vi "Call_signal_fromHW.vi"(5 "Plot window":string) -> (1 "Selected signals":string[](array[string]), 2 "Ready?":bool)   [LabVIEW 2022 SP3]
doc: "Through this function you can select the stored signals from the Main_menu."
panel:
  in  "Working Path":path
  in  "Load Signals profile":bool
  in  "Save Signals profile":bool
  in  "Select signals":i32[](listbox)
  out "Clone Name":string
  in  "Add to graph":bool
  # "First Save Signals before\nto load Signals"
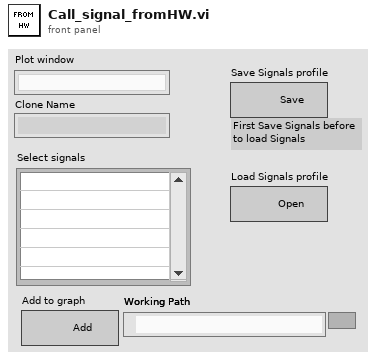
[diagram p1: front panel]
types:
  T1 = enum32{"Invalid", "Standard", "Closed", "Hidden", "Minimized", "Maximized"}
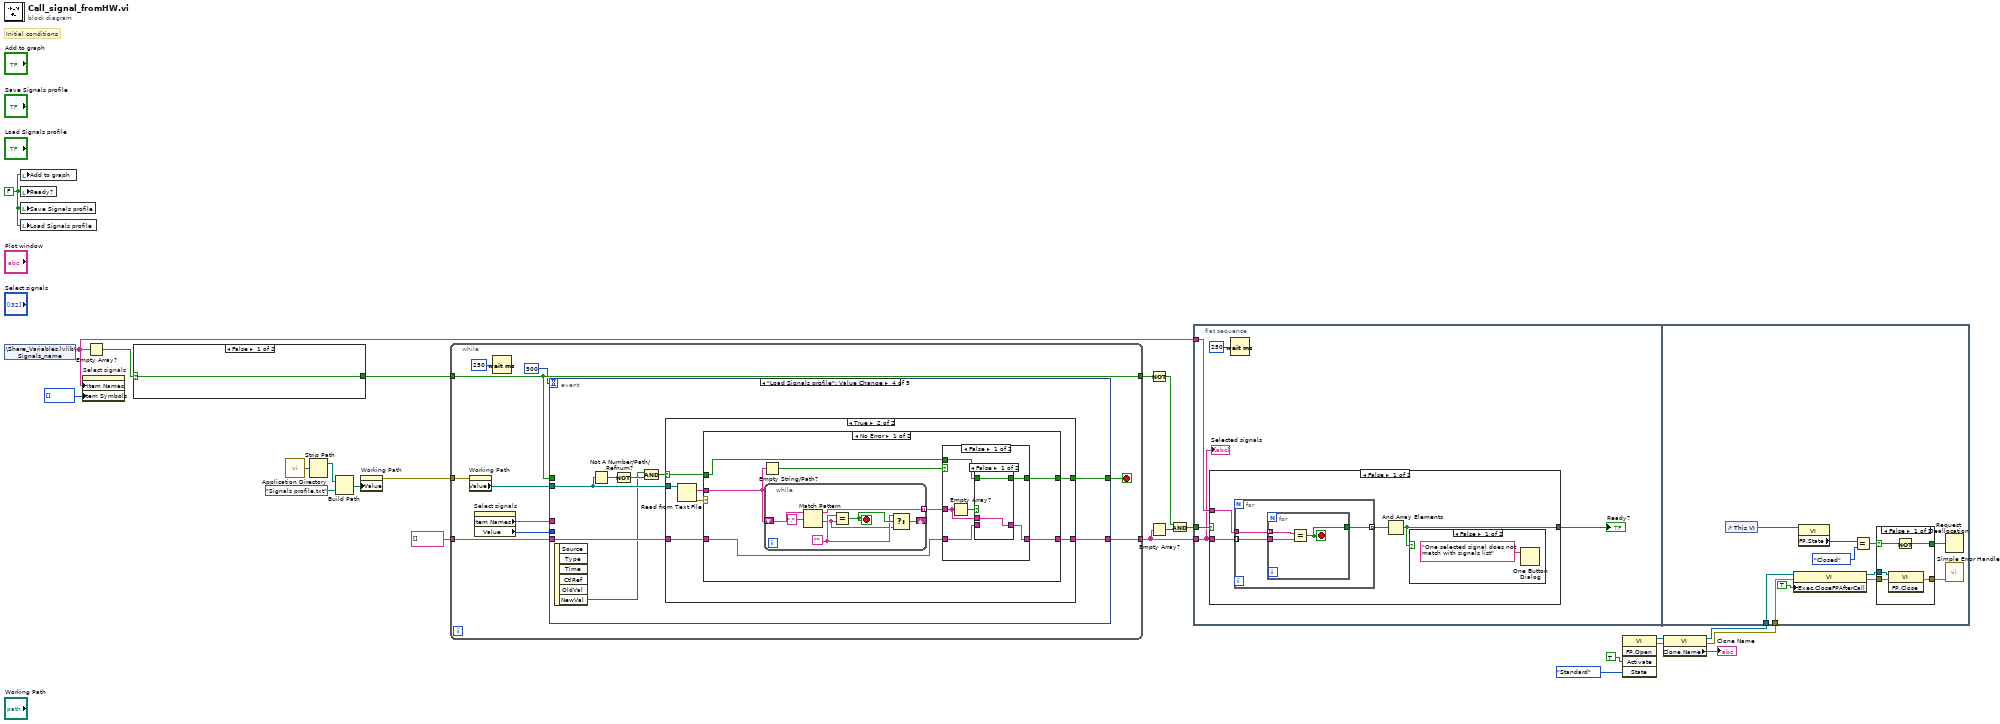
[diagram p0: block diagram]
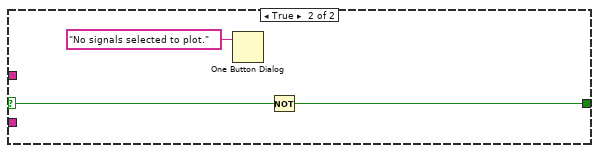
[diagram p3: hidden frame]
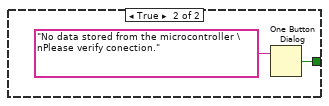
[diagram p5: hidden frame]
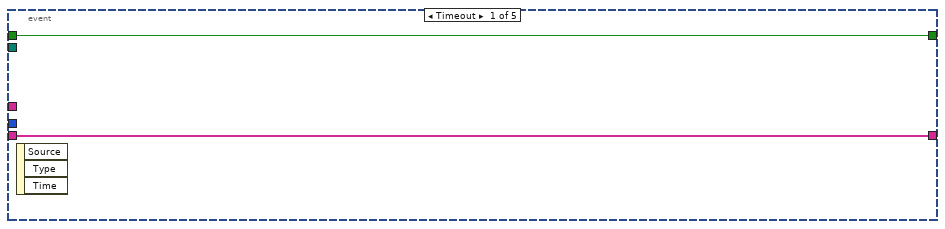
[diagram p6: hidden frame]
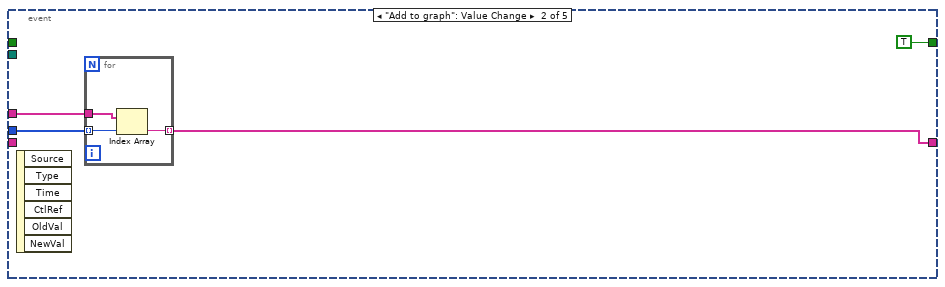
[diagram p7: hidden frame]
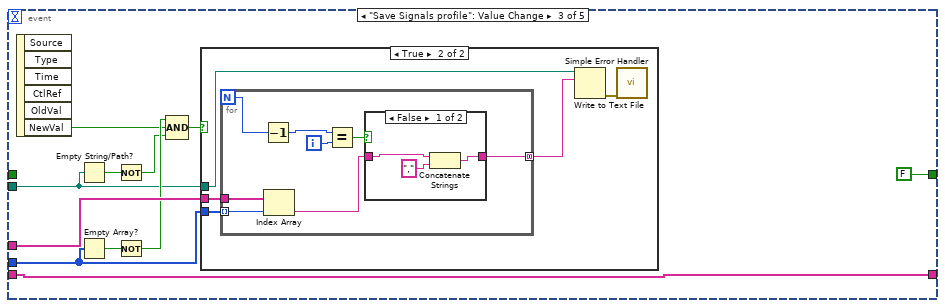
[diagram p8: hidden frame]
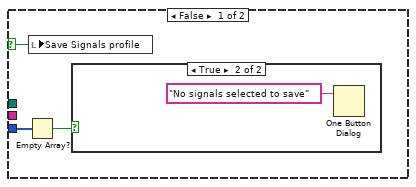
[diagram p9: hidden frame]
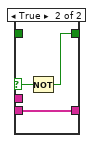
[diagram p13: hidden frame]
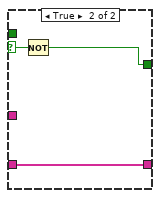
[diagram p14: hidden frame]
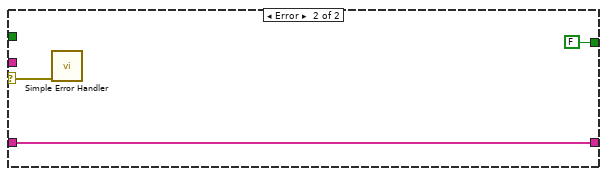
[diagram p15: hidden frame]
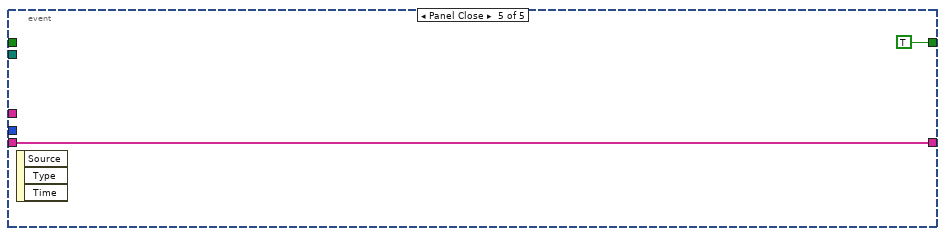
[diagram p16: hidden frame]
diagram:
  w13 = FALSE
  # "Initial conditions"
  n1 = shared-variable ".\\Share_Variables.lvlib\\Signals_name"() -> (w4:string[])  [unwired: 1 in, 1 out]
  n2 = local write "Add to graph"(w13) -> ()
  n3 = local write "Ready?"(w13) -> ()
  n4 = local write "Save Signals profile"(w13) -> ()
  n5 = local write "Load Signals profile"(w13) -> ()
  n6 = property on="Select signals" class="LstBox (strict)"("Item Names"=w4, "Item Symbols"=i32[] []) -> ()  [unwired: 2 in, 2 out]
  n7 = Empty Array?(array=w4) -> (empty?=w19:bool)
  n8 = case shown="False" w19 {
    selector: w19 -> [w24 _]
    tunnel: [w24 w25] -> w18
    frame False {
    }
    frame True {
      n9 = One Button Dialog(message="No data stored from the microcontroller \nPlease verify conection.") -> (true=w25:bool)  [unwired: 1 in]
    }
  }
  n10 = call <vilib>:"Application Directory.vi"() -> ("Application Directory"=w11:path)
  n11 = Strip Path(path=w11) -> (stripped path=w12:path)  [unwired: 1 out]
  n12 = Build Path(base path=w12, name or relative path=path "Signals profile.txt" ("default name")) -> (appended path=w7:path)
  n13 = property on="Working Path" class="Path"("Value"=w7) -> (error out=w6:errorcluster)  [unwired: 2 in, 1 out]
  n14 = while {
    tunnel: w18 -> [w32]
    tunnel: [w36] -> w1
    tunnel: string[] [] -> [w35]
    tunnel: [w32] -> w10
    tunnel: w6 -> [w29]
    stop <- w31 stop-if-true
    n15 = property on="Working Path" class="Path"(error in=w29) -> ("Value"=w28:path)  [unwired: 1 in, 2 out]
    n16 = property on="Select signals" class="LstBox (strict)"() -> ("Item Names"=w34:string[], "Value"=w33:i32[])  [unwired: 2 in, 2 out]
    n17 = Wait (ms)(milliseconds to wait=u32 250) -> ()  [unwired: 1 out]
    n18 = event shown="[3] \"Load Signals profile\": Value Change" {
      selector: _ -> [_ _ _ _ _]
      dyn-events: _ -> [_ _ _ _ _]
      timeout: 500 -> [_ _ _ _ _]
      tunnel: [w37 TRUE FALSE ("true") w84 TRUE] -> w31
      tunnel: [w38 w40 w54 w85 w126] -> w36
      tunnel: w35 -> [w38 _ w54 w83 w126]
      tunnel: w34 -> [_ w42 w55 _ _]
      tunnel: w33 -> [_ w41 w53 _ _]
      tunnel: w28 -> [_ _ w46 w82 _]
      tunnel: w32 -> [w37 _ _ _ _]
      event Timeout {
        n19 = event-data() -> ()  [unwired: 1 in, 3 out]
      }
      event "Add to graph": Value Change {
        n20 = event-data() -> ()  [unwired: 1 in, 6 out]
        n21 = for {
          tunnel: w41 -> [w45] mode=indexing
          tunnel: [w44] -> w40 mode=indexing
          tunnel: w42 -> [w43]
          n22 = Index Array(array=w43, index=w45) -> (element=w44:string)
        }
      }
      event "Save Signals profile": Value Change {
        n23 = event-data() -> ("NewVal"=w49:bool)  [unwired: 1 in, 5 out]
        n24 = Empty String/Path?(string/path=w46) -> (empty?=w51:bool)
        n25 = Empty Array?(array=w53) -> (empty?=w52:bool)
        n26 = Not(x=w51) -> (.not. x?=w48:bool)
        n27 = Not(x=w52) -> (.not. x?=w50:bool)
        n28 = Compound Arithmetic op=AND(w50, w49, w48) -> (w47:bool)
        n29 = case shown="True" w47 {
          selector: w47 -> [w57 _]
          tunnel: w55 -> [_ w62]
          tunnel: w53 -> [w59 w63]
          tunnel: w46 -> [_ w65]
          frame False {
            n30 = Empty Array?(array=w59) -> (empty?=w58:bool)
            n31 = local write "Save Signals profile"(w57) -> ()
            n32 = case shown="True" w58 {
              frame False {
              }
              frame True {
                n33 = One Button Dialog(message="No signals selected to save") -> ()  [unwired: 1 in, 1 out]
              }
            }
          }
          frame True {
            n34 = for {
              N -> [w71]
              tunnel: w63 -> [w73] mode=indexing
              tunnel: w62 -> [w72]
              tunnel: [w66] -> w61 mode=concatenating
              i -> [w69]
              n35 = Decrement(x=w71) -> (x-1=w70:i32)
              n36 = Index Array(array=w72, index=w73) -> (element=w67:string)
              n37 = Equal?(x=w70, y=w69) -> (x = y?=w68:bool)
              n38 = case shown="False" w68 {
                tunnel: w67 -> [w76 w77]
                tunnel: [w75 w77] -> w66
                frame False {
                  n39 = Concatenate Strings(w76, ",") -> (w75:string)
                }
                frame True {
                }
              }
            }
            n40 = Write to Text File(file (use dialog)=w65, text=w61) -> (error out=w64:errorcluster)  [unwired: 2 in, 2 out]
            n41 = call <vilib>:"Simple Error Handler.vi"("error in (no error)"=w64) -> ()  [unwired: 4 in, 5 out]
          }
        }
      }
      event "Load Signals profile": Value Change {
        n42 = event-data() -> ("NewVal"=w78:bool)  [unwired: 1 in, 5 out]
        n43 = Not A Number/Path/Refnum?(number/path/refnum=w82) -> (NaN/Path/Refnum?=w81:bool)
        n44 = Not(x=w81) -> (.not. x?=w80:bool)
        n45 = And(x=w78, y=w80) -> (x .and. y?=w79:bool)
        n46 = case shown="True" w79 {
          selector: w79 -> [w87 w91]
          tunnel: [w86 w93] -> w85
          tunnel: [w87 w90] -> w84
          tunnel: w83 -> [w86 w92]
          tunnel: w82 -> [_ w94]
          frame False {
          }
          frame True {
            n47 = Read from Text File(file (use dialog)=w94) -> (text=w89:string, error out=w88:errorcluster)  [unwired: 3 in, 2 out]
            n48 = case shown="No Error" w88 {
              selector: w88 -> [_ w123]
              tunnel: [w100 w125] -> w93
              tunnel: w92 -> [w99 w125]
              tunnel: w91 -> [w98 _]
              tunnel: [w97 FALSE] -> w90
              tunnel: w89 -> [w96 _]
              frame No Error {
                n49 = Empty String/Path?(string/path=w96) -> (empty?=w101:bool)
                n50 = while {
                  shift-right: [w107] -> _
                  shift-left: w96 -> [w105]
                  tunnel: [w103] -> w95 mode=indexing
                  stop <- w108 stop-if-true
                  w106 = ""
                  n51 = Match Pattern(string=w105, regular expression=",") -> (before substring=w103:string, after substring=w104:string)  [unwired: 1 in, 2 out]
                  n52 = Equal?(x=w106, y=w104) -> (x = y?=w108:bool)
                  n53 = Select(t=w106, s=w108, f=w104) -> (s? t:f=w107:string)
                }
                n54 = case shown="False" w101 {
                  selector: w101 -> [_ w121]
                  tunnel: [w112 w122] -> w100
                  tunnel: w99 -> [w111 w122]
                  tunnel: w98 -> [w109 _]
                  tunnel: [w110 w120] -> w97
                  tunnel: w95 -> [w113 _]
                  frame False {
                    n55 = Empty Array?(array=w113) -> (empty?=w114:bool)
                    n56 = case shown="False" w114 {
                      selector: w114 -> [_ w117]
                      tunnel: w113 -> [w116 _]
                      tunnel: [w116 w119] -> w112
                      tunnel: w111 -> [_ w119]
                      tunnel: [w115 w118] -> w110
                      tunnel: w109 -> [w115 _]
                      frame False {
                      }
                      frame True {
                        n57 = Not(x=w117) -> (.not. x?=w118:bool)
                      }
                    }
                  }
                  frame True {
                    n58 = Not(x=w121) -> (.not. x?=w120:bool)
                  }
                }
              }
              frame Error {
                n59 = call <vilib>:"Simple Error Handler.vi"("error in (no error)"=w123) -> ()  [unwired: 4 in, 5 out]
              }
            }
          }
        }
      }
      event Panel Close {
        n60 = event-data() -> ()  [unwired: 1 in, 3 out]
      }
    }
  }
  n61 = Not(x=w10) -> (.not. x?=w5:bool)
  n62 = Empty Array?(array=w1) -> (empty?=w9:bool)
  n63 = And(x=w5, y=w9) -> (x .and. y?=w8:bool)
  n64 = flat-sequence {
    tunnel: w8 -> [w132]
    tunnel: w1 -> [w128]
    tunnel: w4 -> [w131]
    tunnel: w3 -> [w149]
    tunnel: w2 -> [w148]
    frame #0 {
      n65 = case shown="False" w132 {
        selector: w132 -> [_ w145]
        tunnel: w128 -> [w135 _]
        tunnel: w131 -> [w134 _]
        tunnel: [w133 w144] -> w130
        frame False {
          n66 = for {
            tunnel: w135 -> [w139] mode=indexing
            tunnel: w134 -> [w140]
            tunnel: [w138] -> w136 mode=indexing
            n67 = for {
              tunnel: w140 -> [w142] mode=indexing
              tunnel: w139 -> [w143]
              tunnel: [w141] -> w138
              stop <- w141 stop-if-true
              n68 = Equal?(x=w142, y=w143) -> (x = y?=w141:bool)
            }
          }
          n69 = And Array Elements(Boolean array=w136) -> (logical AND=w133:bool)
          n70 = case shown="False" w133 {
            frame False {
              n71 = One Button Dialog(message="One selected signal does not match with signals list") -> ()  [unwired: 1 in, 1 out]
            }
            frame True {
            }
          }
        }
        frame True {
          n72 = One Button Dialog(message="No signals selected to plot.") -> ()  [unwired: 1 in, 1 out]
          n73 = Not(x=w145) -> (.not. x?=w144:bool)
        }
      }
      "Ready?" <- w130
      n74 = Wait (ms)(milliseconds to wait=u32 250) -> ()  [unwired: 1 out]
      "Selected signals" <- w128
    }
    frame #1 {
      n75 = control-ref of="This VI"() -> (w156:refnum<vi>)
      n76 = property class="VI"(reference=w149, error in=w148, "Exec.CloseFPAfterCall"=TRUE ("Activate?")) -> (reference out=w151:refnum<vi>, error out=w152:errorcluster)
      n77 = property class="VI"(reference=w156) -> ("FP.State"=w155:T1)  [unwired: 1 in, 2 out]
      n78 = Equal?(x=w155, y=T1."Closed" ("Front Panel Window:State")) -> (x = y?=w157:bool)
      n79 = case shown="False" w157 {
        selector: w157 -> [w159 w163]
        tunnel: [w162 w164] -> w153
        tunnel: w151 -> [w161 _]
        tunnel: w152 -> [w160 w164]
        tunnel: [w158 w163] -> w154
        frame False {
          n80 = invoke class="VI" method="FP.Close"(reference=w161, error in=w160) -> (error out=w162:errorcluster)  [unwired: 1 in, 2 out]
          n81 = Not(x=w159) -> (.not. x?=w158:bool)
        }
        frame True {
        }
      }
      n82 = Request Deallocation(w154) -> ()
      n83 = call <vilib>:"Simple Error Handler.vi"("error in (no error)"=w153) -> ()  [unwired: 4 in, 5 out]
    }
  }
  n84 = invoke on="Invoke Node" class="VI" method="FP.Open"("Activate"=TRUE ("Activate?"), "State"=T1."Standard") -> (reference out=w21:refnum<vi>, error out=w22:errorcluster)  [unwired: 3 in, 3 out]
  n85 = property on="Property Node" class="VI"(reference=w21, error in=w22) -> (reference out=w3:refnum<vi>, error out=w2:errorcluster, "Clone Name"=→"Clone Name":string)
